vi "选题序号.vi"(3 "题目总数":dbl) -> (1 "添加的数组":string[](array[string]), 2 "布尔":bool)   [LabVIEW 2014]
panel:
  out "x*y":dbl
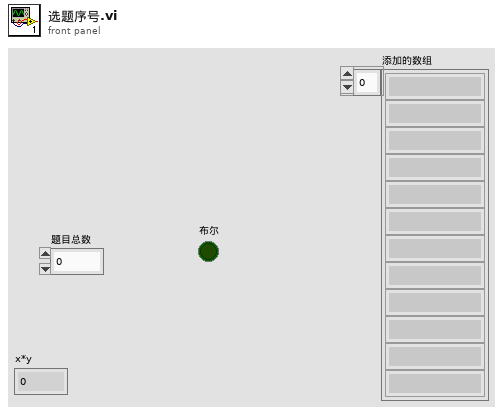
[diagram p1: front panel]
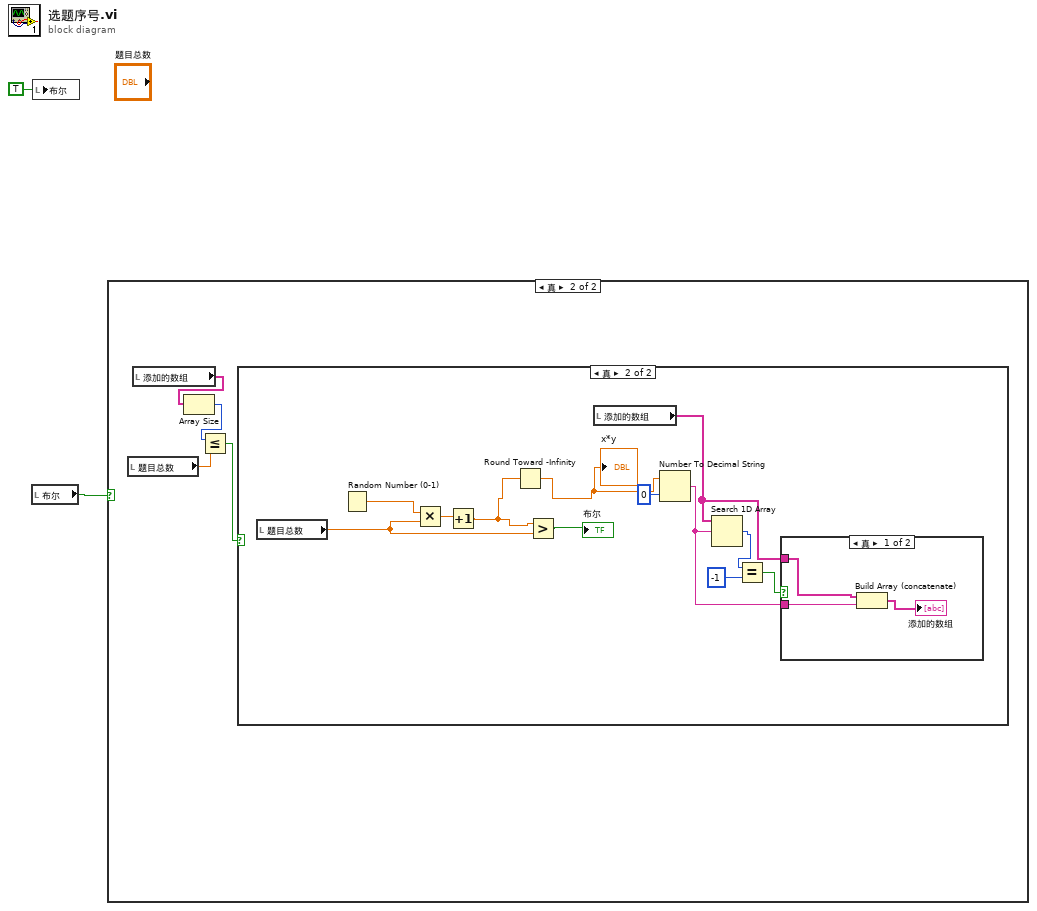
[diagram p0: block diagram]
diagram:
  n1 = local read "布尔"() -> (w1:bool)
  n2 = local write "布尔"(TRUE ("布尔")) -> ()
  n3 = case shown="真" w1 {
    frame False {
    }
    frame True {
      n4 = local read "题目总数"() -> (w4:dbl)
      n5 = local read "添加的数组"() -> (w6:string[])
      n6 = Array Size(array=w6) -> (size(s)=w5:i32)
      n7 = Less Or Equal?(x=w5, y=w4) -> (x <= y?=w3:bool)
      n8 = case shown="真" w3 {
        frame False {
        }
        frame True {
          n9 = local read "题目总数"() -> (w18:dbl)
          n10 = Random Number (0-1)() -> (number: 0 to 1=w17:dbl)
          n11 = Multiply(x=w17, y=w18) -> (x*y=w16:dbl)
          n12 = Increment(x=w16) -> (x+1=w8:dbl)
          n13 = Round Toward -Infinity(1:w8) -> (0:w7:dbl)
          "x*y" <- w7
          n14 = Greater?(x=w8, y=w18) -> (0:→"布尔":bool)
          n15 = local read "添加的数组"() -> (w9:string[])
          n16 = Number To Decimal String(number=w7, width (-)=i16 0 ("宽度(-)")) -> (decimal integer string=w13:string)
          n17 = Search 1D Array(1D array=w9, element=w13) -> (index of element=w12:i32)  [unwired: 1 in]
          n18 = Equal?(x=w12, y=-1) -> (x = y?=w10:bool)
          n19 = case shown="真" w10 {
            tunnel: w13 -> [w21 _]
            tunnel: w9 -> [w19 _]
            frame True {
              n20 = Build Array (concatenate)(w19, w21) -> (→"添加的数组":string[])
            }
            frame False {
            }
          }
        }
      }
    }
  }
